vi "SR830KepcoMagnetController.vi"(5 "Field dwell time (ms)":u32=50, 6 "Zero Field Wait (s)":u32=60, 7 "Field Step size (mT)":dbl=0.05, 8 "error in (no error)":errorcluster, 9 "Target Field (mT)":dbl, 10 "Aux Channel (1: Channel 1)":u16(ring)=1 items=["Channel 1"=1, "Channel 2"=2, "Channel 3"=3, "Channel 4"=4], 11 "VISA resource name":refnum<visa-resource-name>="SR830LockIn2") -> (0 "error out":errorcluster, 1 "Final Field (mT)":dbl=0.016400000000000192, 2 "Start Field (mT)":dbl=-1.0335999999999999, 3 "VISA resource name out":refnum<visa-resource-name>="SR830LockIn2")   [LabVIEW 2016]
uses:
  <instrlib>/Stanford Research 830/Stanford Research 830.lvlib
panel:
  # "This VI uses the Aux Out of the SR830 to control the magnetic field via Current control.\nChoose either Aux Out 1 or Aux out 2 as the control channel\nDefault to Channel 1"
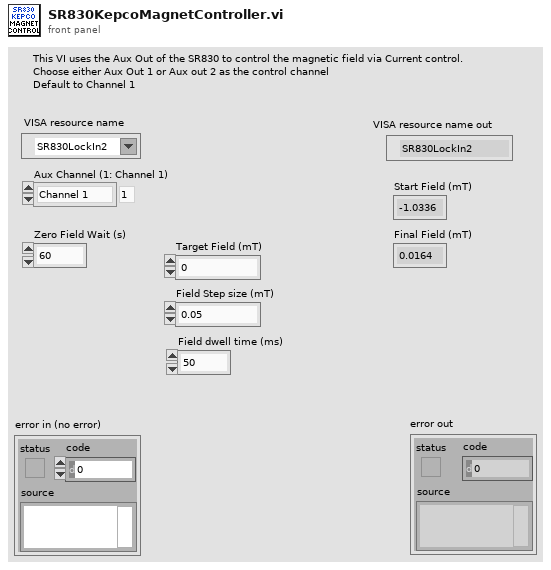
[diagram p1: front panel]
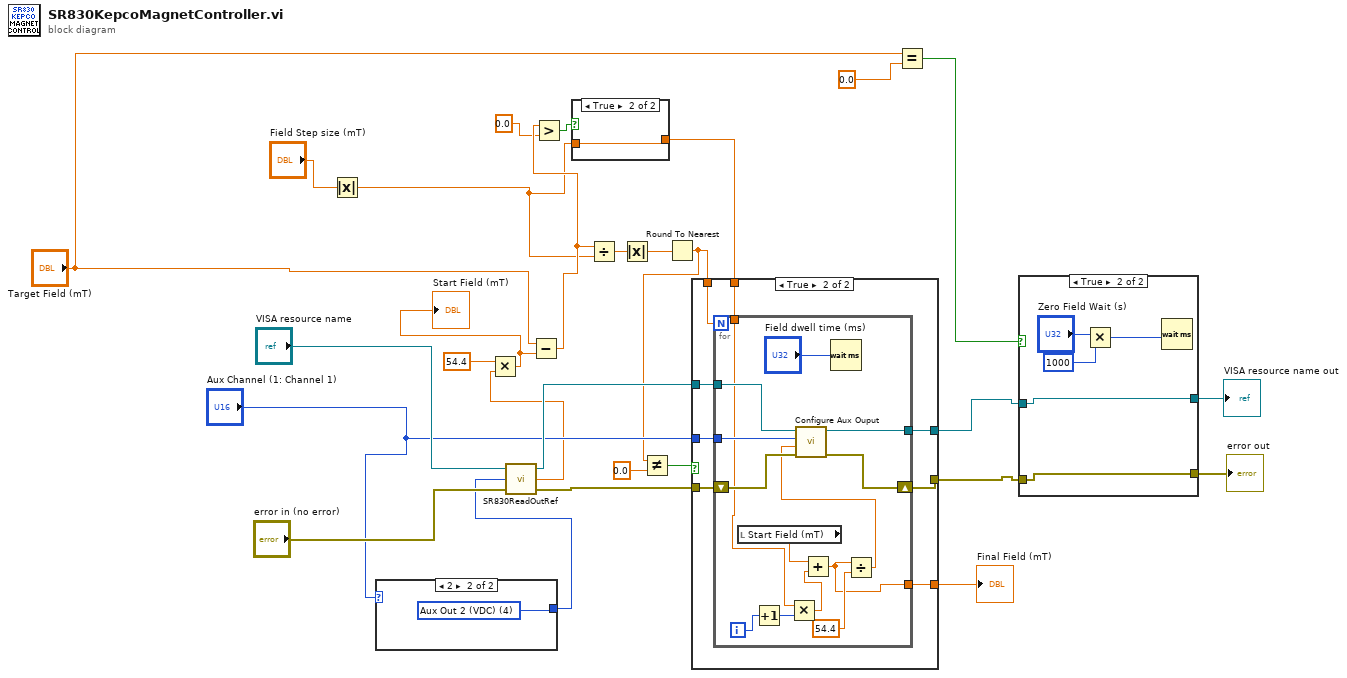
[diagram p0: block diagram]
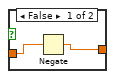
[diagram p3: hidden frame]
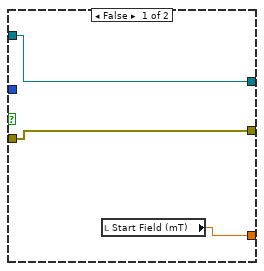
[diagram p4: hidden frame]
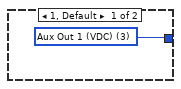
[diagram p5: hidden frame]
diagram:
  n1 = Absolute Value(x="Field Step size (mT)") -> (abs(x)=w10:dbl)
  n2 = case shown="2" "Aux Channel (1: Channel 1)" {
    tunnel: [w29 w30] -> w23
    frame 1, Default {
      w29 = u16 3 items=["Voltage Out (Vrms)"=1, "Frequency (Hz)"=2, "Aux Out 1 (VDC)"=3, "Aux Out 2 (VDC)"=4, "Time Constant (s)"=5] ("ReadOut (1: Voltage Amplitude)")
    }
    frame 2 {
      w30 = u16 4 items=["Voltage Out (Vrms)"=1, "Frequency (Hz)"=2, "Aux Out 1 (VDC)"=3, "Aux Out 2 (VDC)"=4, "Time Constant (s)"=5, "Roll-Off Slope (dB/oct)"=6] ("ReadOut (1: Voltage Amplitude)")
    }
  }
  n3 = call "SR830ReadOutRef.vi"("error in (no error)"="error in (no error)", "ReadOut (1: Voltage Amplitude)"=w23, "VISA resource name"="VISA resource name") -> ("error out"=w25:errorcluster, "ReadOut"=w22:dbl, "VISA resource name out"=w26:refnum<visa-resource-name>)
  n4 = Multiply(x=54.4, y=w22) -> (x*y=w20:dbl)
  "Start Field (mT)" <- w20
  n5 = Subtract(x="Target Field (mT)", y=w20) -> (x-y=w13:dbl)
  n6 = Greater?(x=w13, y=0.0) -> (0:w11:bool)
  n7 = case shown="True" w11 {
    tunnel: w10 -> [w32 w33]
    tunnel: [w31 w33] -> w9
    frame False {
      n8 = Negate(x=w32) -> (-x=w31:dbl)
    }
    frame True {
    }
  }
  n9 = Divide(x=w13, y=w10) -> (x/y=w18:dbl)
  n10 = Absolute Value(x=w18) -> (abs(x)=w17:dbl)
  n11 = Round To Nearest(number=w17) -> (nearest integer value=w14:dbl)
  n12 = Not Equal?(x=w14, y=0.0) -> (x != y?=w16:bool)
  n13 = case shown="True" w16 {
    tunnel: [w36 w44] -> w4
    tunnel: [w35 w43] -> w2
    tunnel: w26 -> [w36 w42]
    tunnel: w25 -> [w35 w41]
    tunnel: "Aux Channel (1: Channel 1)" -> [_ w40]
    tunnel: w14 -> [_ w39]
    tunnel: w9 -> [_ w38]
    tunnel: [w34 w37] -> w8
    frame False {
      n14 = local read "Start Field (mT)"() -> (w34:dbl)
    }
    frame True {
      n15 = for {
        N: w39 -> [_]
        tunnel: w40 -> [w58]
        shift-right: [w54] -> w43
        shift-left: w41 -> [w56]
        tunnel: w42 -> [w57]
        tunnel: [w55] -> w44
        tunnel: w38 -> [w50]
        tunnel: [w45] -> w37
        i -> [w53]
        n16 = local read "Start Field (mT)"() -> (w52:dbl)
        n17 = Increment(x=w53) -> (x+1=w51:i32)
        n18 = Multiply(x=w50, y=w51) -> (x*y=w49:dbl)
        n19 = Add(x=w52, y=w49) -> (x+y=w45:dbl)
        n20 = Wait (ms)(milliseconds to wait="Field dwell time (ms)") -> ()  [unwired: 1 out]
        n21 = Divide(x=w45, y=54.4) -> (x/y=w47:dbl)
        n22 = call <instrlib>:"Configure Aux Ouput.vi"("error in (no error)"=w56, "Aux Output Voltage (1 V)"=w47, "Aux Channel (1: Channel 1)"=w58, "VISA resource name"=w57) -> ("error out"=w54:errorcluster, "VISA resource name out"=w55:refnum<visa-resource-name>)  [unwired: 6 in]
      }
    }
  }
  "Final Field (mT)" <- w8
  n23 = Equal?(x="Target Field (mT)", y=0.0) -> (x = y?=w7:bool)
  n24 = case shown="True" w7 {
    tunnel: w4 -> [w60 w62]
    tunnel: [w60 w62] -> w3
    tunnel: w2 -> [w59 w61]
    tunnel: [w59 w61] -> w1
    frame False {
    }
    frame True {
      n25 = Multiply(x="Zero Field Wait (s)", y=u32 1000) -> (x*y=w63:u32)
      n26 = Wait (ms)(milliseconds to wait=w63) -> ()  [unwired: 1 out]
    }
  }
  "VISA resource name out" <- w3
  "error out" <- w1
